vi "Vision Test 2.vi"(7 "error in":errorcluster) -> (20 "Matches (Geometric Matching 1)":T2[](array[typedef]) {"Correlation Score" format="%.2f"; "Target Template Curve Score" format="%.2f"; "Template Target Curve Score" format="%.2f"; "Bounding Box"."y" format="%.2f"; "Bounding Box"."x" format="%.2f"; "Position"."y" format="%.2f"; "Position"."x" format="%.2f"; "Score" format="%.2f"; "Scale" format="%.2f"; "Angle" format="%.2f"; "Occlusion %" format="%.2f"}, 21 "Calibrated Matches (Geometric Matching 1)":T2[](array[typedef]) {"Correlation Score" format="%.2f"; "Target Template Curve Score" format="%.2f"; "Template Target Curve Score" format="%.2f"; "Bounding Box"."y" format="%.2f"; "Bounding Box"."x" format="%.2f"; "Position"."y" format="%.2f"; "Position"."x" format="%.2f"; "Score" format="%.2f"; "Scale" format="%.2f"; "Angle" format="%.2f"; "Occlusion %" format="%.2f"}, 22 "Number of Matches (Geometric Matching 1)":i32, 27 "error out":errorcluster)   [LabVIEW 2015]
uses:
  <vilib>/vision/Pattern Matching.llb/IMAQ GM Match Report.ctl
  <vilib>/vision/Pattern Matching.llb/IMAQ Curve Parameters.ctl
  <vilib>/vision/Pattern Matching.llb/IMAQ Match Range Setting.ctl
  <vilib>/vision/driver/NI_Vision_Acquisition_Software.lvlib
  <vilib>/vision/NI_Vision_Development_Module.lvlib
panel:
  out "Image Out":T1(plugin-control)
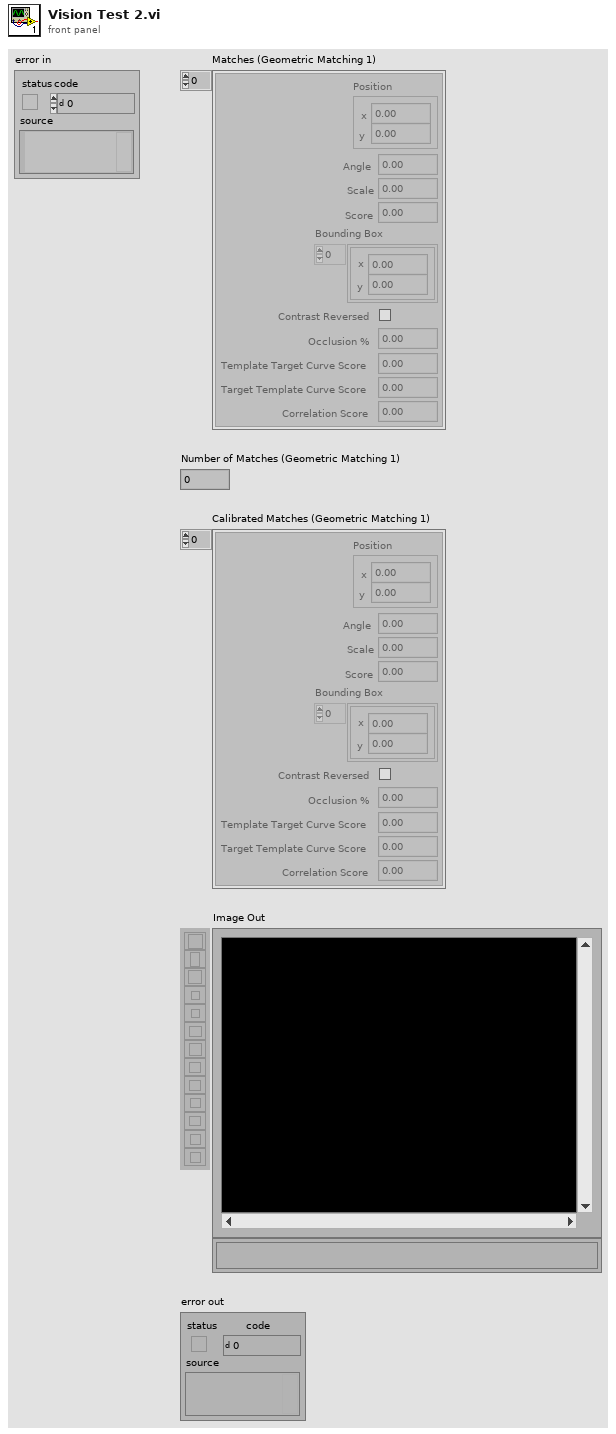
[diagram p1: front panel]
types:
  T1 = typedef "IMAQ Image.ctl" = refnum<image>
  T2 = typedef "IMAQ GM Match Report.ctl" = cluster{"Position":cluster{"x":sgl, "y":sgl}, "Angle":sgl, "Scale":sgl, "Score":sgl, "Bounding Box":cluster{"x":sgl, "y":sgl}[], "Contrast Reversed":bool, "Occlusion %":sgl, "Template Target Curve Score":sgl, "Target Template Curve Score":sgl, "Correlation Score":sgl}
  T3 = typedef "IMAQ Curve Parameters.ctl" = cluster{"Extraction Mode":u32, "Edge Threshold":i32, "Edge Filter Size":u32, "Min Length":i32, "Row Search Step Size":i32, "Col Search Step Size":i32, "Max Endpoint Gap":i32, "Closed":bool, "Subpixel":bool}
  T4 = typedef "IMAQ Match Range Setting.ctl" = cluster{"Match Constraints":u32, "Min":dbl, "Max":dbl}
  T5 = cluster{"Curve Parameters":T3, "Match Mode":cluster{"Rotation":bool, "Scale":bool, "Occlusion":bool, "Reserved":bool, "Reserved":bool, "Reserved":bool}, "Range Settings":T4[], "Number of Matches":i32, "Minimum Match Score":sgl, "SubPixel Accuracy":bool, "Adv. Geometric Match Options 2":cluster{"Setup Data Item":u16, "Item Value":dbl}[]}
  T6 = cluster{"Global Rectangle":i32[], "Contours":cluster{"ID":enum32{"External", "Internal"}, "Type":u32, "Coordinates":i32[]}[]}
  T7 = enum32{"AutoM", "Close", "Dilate", "Erode", "Gradient", "Gradient in", "Gradient out", "HitMiss", "Open", "PClose", "POpen", "Thick", "Thin"}
  T8 = typedef "IMAQdx.ctl" = refnum<k21>
  T9 = cluster{"histogram":u32[], "Minimal Value":sgl, "Maximal Value":sgl, "Starting Value":sgl, "Interval Width":sgl, "Mean Value":sgl, "Standard  Variation":sgl, "Area (pixels)":i32}
  T10 = typedef "Image Type" = u32
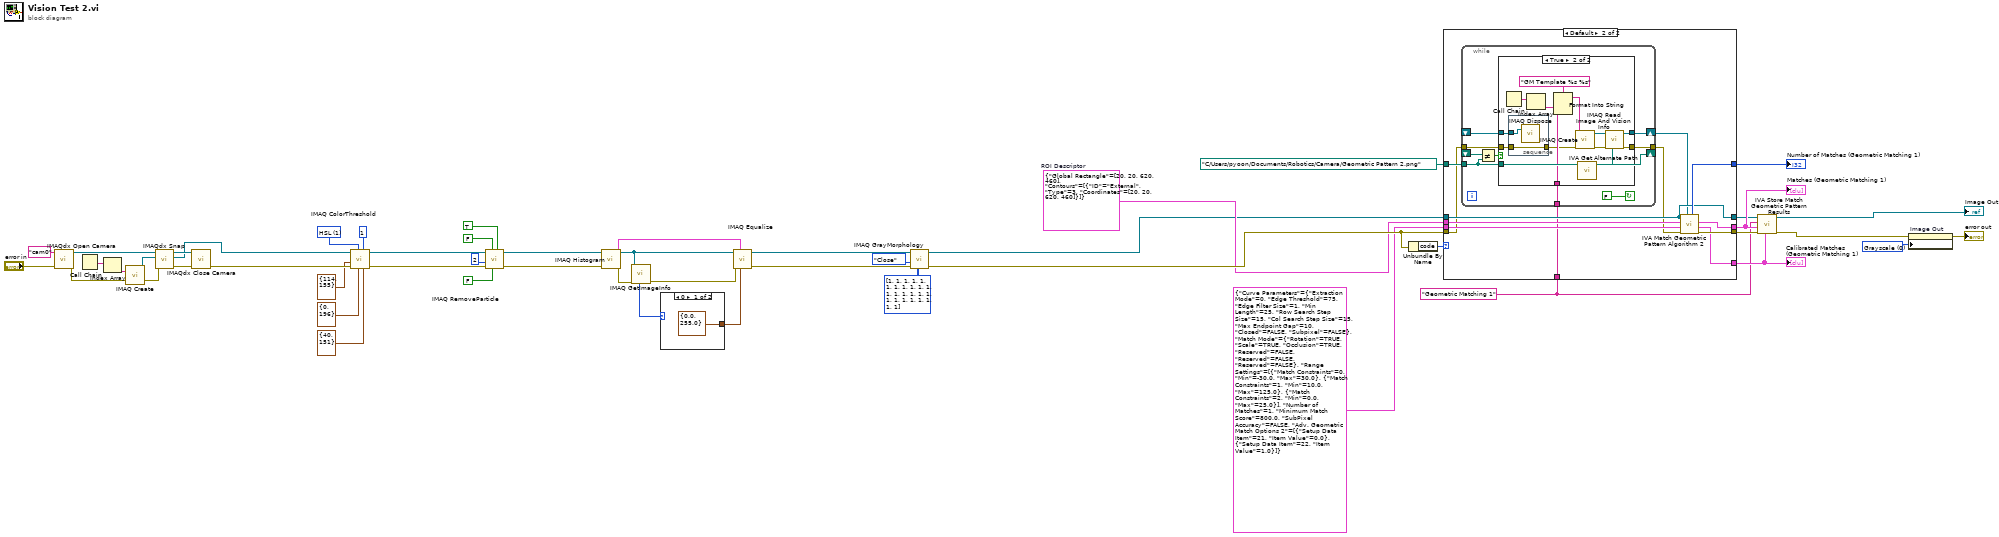
[diagram p0: block diagram]
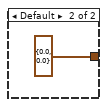
[diagram p4: hidden frame]
diagram:
  w1 = u32 0 items=["Grayscale", "Binary", "Gradient", "Rainbow", "Temperature", "User Defined", "Binary 16 Bit", "Gradient 16 Bit", "Rainbow 16 Bit", "Temperature 16 Bit", "User Defined 16 Bit"] ("Palette Type")
  w4 = "Geometric Matching 1" ("Step Name")
  w14 = T6 {"Global Rectangle"=[20, 20, 620, 460], "Contours"=[{"ID"=enum."External", "Type"=3, "Coordinates"=[20, 20, 620, 460]}]}  # ROI Descriptor
  w38 = u16 1 items=["RGB", "HSL", "HSV", "HSI"] ("Color Mode")
  n1 = call <vilib>:"IMAQdx Open Camera.vi"("error in"="error in", "Session In"="cam0" ("Interface Name")) -> ("error out"=w49:errorcluster, "Session Out"=w43:T8)  [unwired: 1 in, 7 out]
  n2 = Call Chain() -> (call chain=w41:string[])
  n3 = Index Array(array=w41) -> (element=w40:string)  [unwired: 1 in]
  n4 = call "IMAQ Create"("Image Name"=w40, "error in (no error)"=w49) -> ("New Image"=w45:T1, "error out"=w44:errorcluster)  [unwired: 2 in, 1 out]
  n5 = call <vilib>:"IMAQdx Snap.vi"("error in"=w44, "Image In"=w45, "Session In"=w43) -> ("error out"=w47:errorcluster, "Image Out"=w34:T1, "Session Out"=w48:T8)  [unwired: 6 out]
  n6 = call <vilib>:"IMAQdx Close Camera.vi"("error in"=w47, "Session In"=w48) -> ("error out"=w46:errorcluster)  [unwired: 9 out]
  n7 = call "IMAQ ColorThreshold"("Blue or Luma or Val or Inten Range"=cluster{"Lower value":i32, "Upper value":i32} {"Lower value"=40, "Upper value"=151}, "Replace Value"=1, "Green or Sat Range"=cluster{"Lower value":i32, "Upper value":i32} {"Lower value"=0, "Upper value"=196}, "Color Mode"=w38, "error in (no error)"=w46, "Red or Hue Range"=cluster{"Lower value":i32, "Upper value":i32} {"Lower value"=114, "Upper value"=155}, "Image Src"=w34) -> ("error out"=w33:errorcluster, "Image Dst Out"=w28:T1)  [unwired: 1 in, 2 out]
  n8 = call "IMAQ RemoveParticle"("Connectivity 4/8 (8)"=TRUE, "Low Pass/High Pass (Low)"=FALSE, "Square/Hexa (Square)"=FALSE, "error in (no error)"=w33, "Number of Erosion"=2, "Image Src"=w28) -> ("error out"=w27:errorcluster, "Image Dst Out"=w23:T1)  [unwired: 1 in, 3 out]
  n9 = call "IMAQ Histogram"("error in (no error)"=w27, "Image"=w23) -> ("error out"=w22:errorcluster, "Histogram Report"=w25:T9)  [unwired: 3 in, 5 out]
  n10 = call "IMAQ GetImageInfo"("error in (no error)"=w22, "Image"=w23) -> ("error out"=w21:errorcluster, "Image Type"=w24:T10)  [unwired: 8 out]
  n11 = case shown="0" w24 {
    tunnel: [cluster{"Minimum":sgl, "Maximum":sgl} {"Minimum"=0.0, "Maximum"=255.0} ("Range") cluster{"Minimum":sgl, "Maximum":sgl} {"Minimum"=0.0, "Maximum"=0.0} ("Range")] -> w20
    frame 0 {
    }
    frame Default {
    }
  }
  n12 = call "IMAQ Equalize"("Range"=w20, "Histogram Report"=w25, "error in (no error)"=w21, "Image Src"=w23) -> ("error out"=w26:errorcluster, "Image Dst Out"=w17:T1)  [unwired: 2 in, 4 out]
  n13 = call "IMAQ GrayMorphology"("Structuring Element"=i32[][] [[1, 1, 1, 1, 1], [1, 1, 1, 1, 1], [1, 1, 1, 1, 1], [1, 1, 1, 1, 1], [1, 1, 1, 1, 1]], "error in (no error)"=w26, "Operation"=T7."Close", "Image Src"=w17) -> ("error out"=w16:errorcluster, "Image Dst Out"=w13:T1)  [unwired: 3 in, 3 out]
  n14 = Unbundle By Name(w16) -> ("code"=w7:i32)
  n15 = case shown="Default" w7 {
    tunnel: path "C:/Users/pyoon/Documents/Robotics/Camera/Geometric Pattern 2.png" ("Template File Path") -> [_ w58]
    tunnel: w16 -> [_ w57]
    tunnel: T5 {"Curve Parameters"={"Extraction Mode"=0, "Edge Threshold"=75, "Edge Filter Size"=1, "Min Length"=25, "Row Search Step Size"=15, "Col Search Step Size"=15, "Max Endpoint Gap"=10, "Closed"=FALSE, "Subpixel"=FALSE}, "Match Mode"={"Rotation"=TRUE, "Scale"=TRUE, "Occlusion"=TRUE, "Reserved"=FALSE, "Reserved"=FALSE, "Reserved"=FALSE}, "Range Settings"=[{"Match Constraints"=0, "Min"=-30.0, "Max"=30.0}, {"Match Constraints"=1, "Min"=10.0, "Max"=125.0}, {"Match Constraints"=2, "Min"=0.0, "Max"=25.0}], "Number of Matches"=1, "Minimum Match Score"=800.0, "SubPixel Accuracy"=FALSE, "Adv. Geometric Match Options 2"=[{"Setup Data Item"=21, "Item Value"=0.0}, {"Setup Data Item"=22, "Item Value"=1.0}]} ("Settings") -> [_ w65]
    tunnel: w14 -> [_ w64]
    tunnel: w13 -> [w53 w59]
    tunnel: [_ w63] -> w12
    tunnel: [_ w62] -> w10
    tunnel: [_ w61] -> w9
    tunnel: [_ w60] -> w8
    tunnel: [w53 w59] -> w6
    tunnel: w4 -> [_ w54]
    frame -1074396199, -1074396198 {
      # "Discard Coordinate System Error"
    }
    frame Default {
      n16 = while {
        shift-right: [w74] -> w55
        shift-left: _ -> [w73]
        tunnel: [w71] -> w56
        tunnel: w57 -> [w70]
        tunnel: w58 -> [w66]
        tunnel: w54 -> [w69]
        shift-right: [w66] -> _
        shift-left: _ -> [w68]
        stop <- FALSE continue-if-true
        n17 = Not Equal?(x=w68, y=w66) -> (x != y?=w67:bool)
        n18 = case shown="True" w67 {
          tunnel: [w76 w88] -> w74
          tunnel: w73 -> [w76 w80]
          tunnel: [w75 w85] -> w71
          tunnel: w70 -> [w75 w81]
          tunnel: w69 -> [_ w82]
          tunnel: w66 -> [_ w78]
          frame False {
          }
          frame True {
            n19 = Call Chain() -> (call chain=w84:string[])
            n20 = stacked-sequence {
              tunnel: w81 -> [w92]
              tunnel: w80 -> [w91]
              tunnel: [w92] -> w79
              frame #0 {
                n21 = call "IMAQ Dispose"("Image"=w91) -> ()  [unwired: 2 in, 4 out]
              }
            }
            n22 = Index Array(array=w84) -> (element=w83:string)  [unwired: 1 in]
            n23 = Format Into String(format string="GM Template %s %s" ("Image Name"), w83, w82) -> (resulting string=w90:string)  [unwired: 2 in, 1 out]
            n24 = call "IMAQ Create"("Image Name"=w90, "error in (no error)"=w79) -> ("New Image"=w87:T1, "error out"=w86:errorcluster)  [unwired: 2 in, 1 out]
            n25 = call <vilib>:"IVA Get Alternate Path.vi"("Path In"=w78) -> ("Path Out"=w77:path)  [unwired: 10 out]
            n26 = call "IMAQ Read Image And Vision Info"("File Path"=w77, "error in (no error)"=w86, "Image"=w87) -> ("error out"=w85:errorcluster, "Image Out"=w88:T1)  [unwired: 1 in, 6 out]
          }
        }
      }
      n27 = call <vilib>:"IVA Match Geometric Pattern Algorithm 2.vi"("Template"=w55, "error in (no error)"=w56, "Settings"=w65, "ROI Descriptor"=w64, "Image"=w59) -> ("error out"=w63:errorcluster, "Calibrated Matches"=w61:T2[], "Matches"=w62:T2[], "Number of Matches"=w60:i32)  [unwired: 1 in, 2 out]
    }
  }
  "Matches (Geometric Matching 1)" <- w10
  "Number of Matches (Geometric Matching 1)" <- w8
  "Calibrated Matches (Geometric Matching 1)" <- w9
  n28 = call <vilib>:"IVA Store Match Geometric Pattern Results.vi"("Calibrated Matches"=w9, "error in (no error)"=w12, "Matches"=w10, "Step Name"=w4, "Image in"=w6) -> ("error out"=w11:errorcluster, "Image dup"=→"Image Out":T1)  [unwired: 5 out]
  n29 = property on="Image Out" class="ImageControl"(error in=w11, "Palette:Palette Type"=w1) -> (error out=→"error out":errorcluster)  [unwired: 1 in, 1 out]
